vi "Select an Actor.vi"(8 "error in":errorcluster, 11 "Actor Store":refnum<class "Actor Store.lvclass">) -> (0 "error out":errorcluster, 1 "Path to Actor":path, 2 "Name of Actor":string, 3 "Actor Store":refnum<class "Actor Store.lvclass">, 4 "Cancelled":bool)   [LabVIEW 2020, in "Add Actor.lvlib"]
uses:
  Add Actor.lvlib
  Localized Strings.vi
  <resource>/dialog/lvconfig.llb/LV Config Write Pathlist.vi
  Classes/Actor Store/Actor Store.lvclass
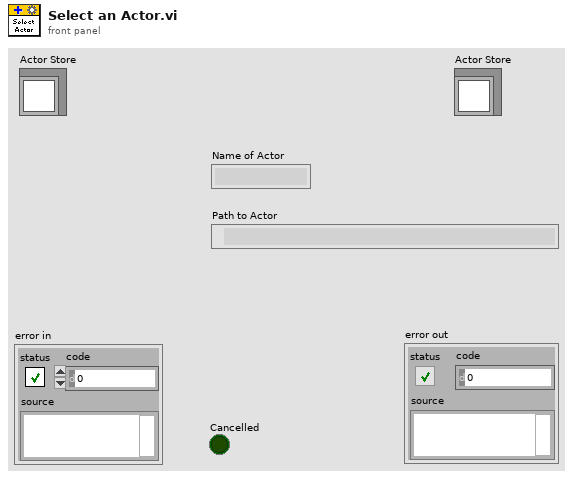
[diagram p1: front panel]
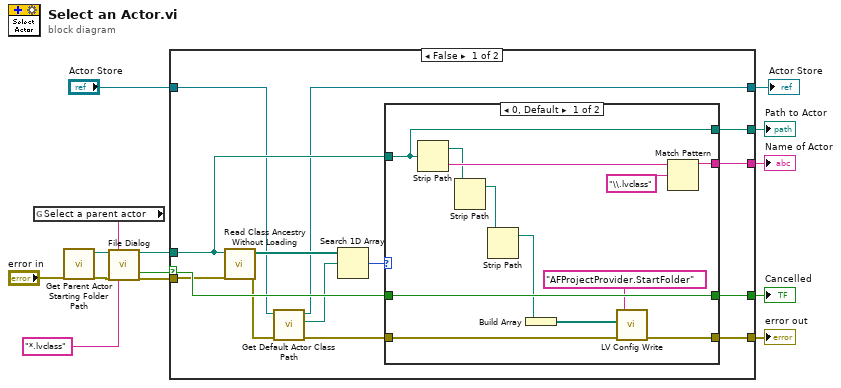
[diagram p0: block diagram]
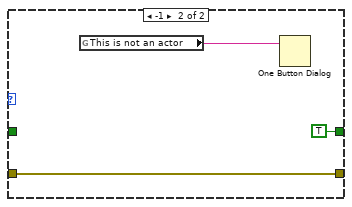
[diagram p2: hidden frame]
diagram:
  n1 = global read "Localized Strings.vi" "Select a parent actor"() -> (w6:string)
  n2 = call "Get Parent Actor Starting Folder Path.vi"("error in (no error)"="error in") -> ("error out"=w3:errorcluster, "Path String"=w5:path)  [unwired: 9 in]
  n3 = call "File Dialog"("start path"=w5, "prompt"=w6, "error in"=w3, "pattern (all files)"="*.lvclass") -> ("selected path"=w12:path, "cancelled"=w11:bool, "error out"=w13:errorcluster)  [unwired: 8 in, 1 out]
  n4 = case shown="False" w11 {
    selector: w11 -> [w26 w46]
    tunnel: w13 -> [w24 w45]
    tunnel: w12 -> [w23 _]
    tunnel: [w28 _] -> w10
    tunnel: [w27 _] -> w9
    tunnel: [w25 w46] -> w8
    tunnel: [w18 w45] -> w7
    tunnel: "Actor Store" -> [w16 w44]
    tunnel: [w15 w44] -> w1
    frame False {
      n5 = call <vilib>:"Read Class Ancestry Without Loading.vi"("error in (no error)"=w24, "LabVIEW Class Path"=w23) -> ("error out"=w20:errorcluster, "Class Ancestry"=w22:path[])  [unwired: 8 in]
      n6 = call "Get Default Actor Class Path.vi"("error in (no error)"=w20, "Actor Store"=w16) -> ("error out"=w19:errorcluster, "Path String"=w17:path, "Actor Store"=w15:refnum<class "Actor Store.lvclass">)  [unwired: 6 in, 1 out]
      n7 = Search 1D Array(1D array=w22, element=w17) -> (index of element=w21:i32)  [unwired: 1 in]
      n8 = case shown="0, Default" w21 {
        tunnel: w23 -> [w37 _]
        tunnel: [w38 _] -> w27
        tunnel: [w37 _] -> w28
        tunnel: w26 -> [w36 _]
        tunnel: [w36 TRUE] -> w25
        tunnel: w19 -> [w34 w41]
        tunnel: [w33 w41] -> w18
        frame 0, Default {
          n9 = Strip Path(path=w37) -> (stripped path=w35:path, name=w40:string)
          n10 = Strip Path(path=w35) -> (stripped path=w30:path)  [unwired: 1 out]
          n11 = Strip Path(path=w30) -> (stripped path=w29:path)  [unwired: 1 out]
          n12 = Build Array(w29) -> (w32:path[])
          n13 = call-poly <resource>:"LV Config Write.vi"("error in (no error)"=w34, "value"=w32, "key"="AFProjectProvider.StartFolder") -> ("error out"=w33:errorcluster)  [unwired: 4 in]
          n14 = Match Pattern(string=w40, regular expression="\\.lvclass") -> (before substring=w38:string)  [unwired: 1 in, 3 out]
        }
        frame -1 {
          n15 = global read "Localized Strings.vi" "This is not an actor"() -> (w42:string)
          n16 = One Button Dialog(message=w42) -> ()  [unwired: 1 in, 1 out]
        }
      }
    }
    frame True {
    }
  }
  "Path to Actor" <- w10
  "Name of Actor" <- w9
  "Cancelled" <- w8
  "error out" <- w7
  "Actor Store" <- w1
